vi "arrayToImage.vi"() -> ()   [LabVIEW 2011]
panel:
  in  "flip axis?":bool
  in  "fringe number":u32
  in  "Boolean":bool
  in  "yPixel":i32
  in  "xPixel":i32
  out "Image":T1(plugin-control)
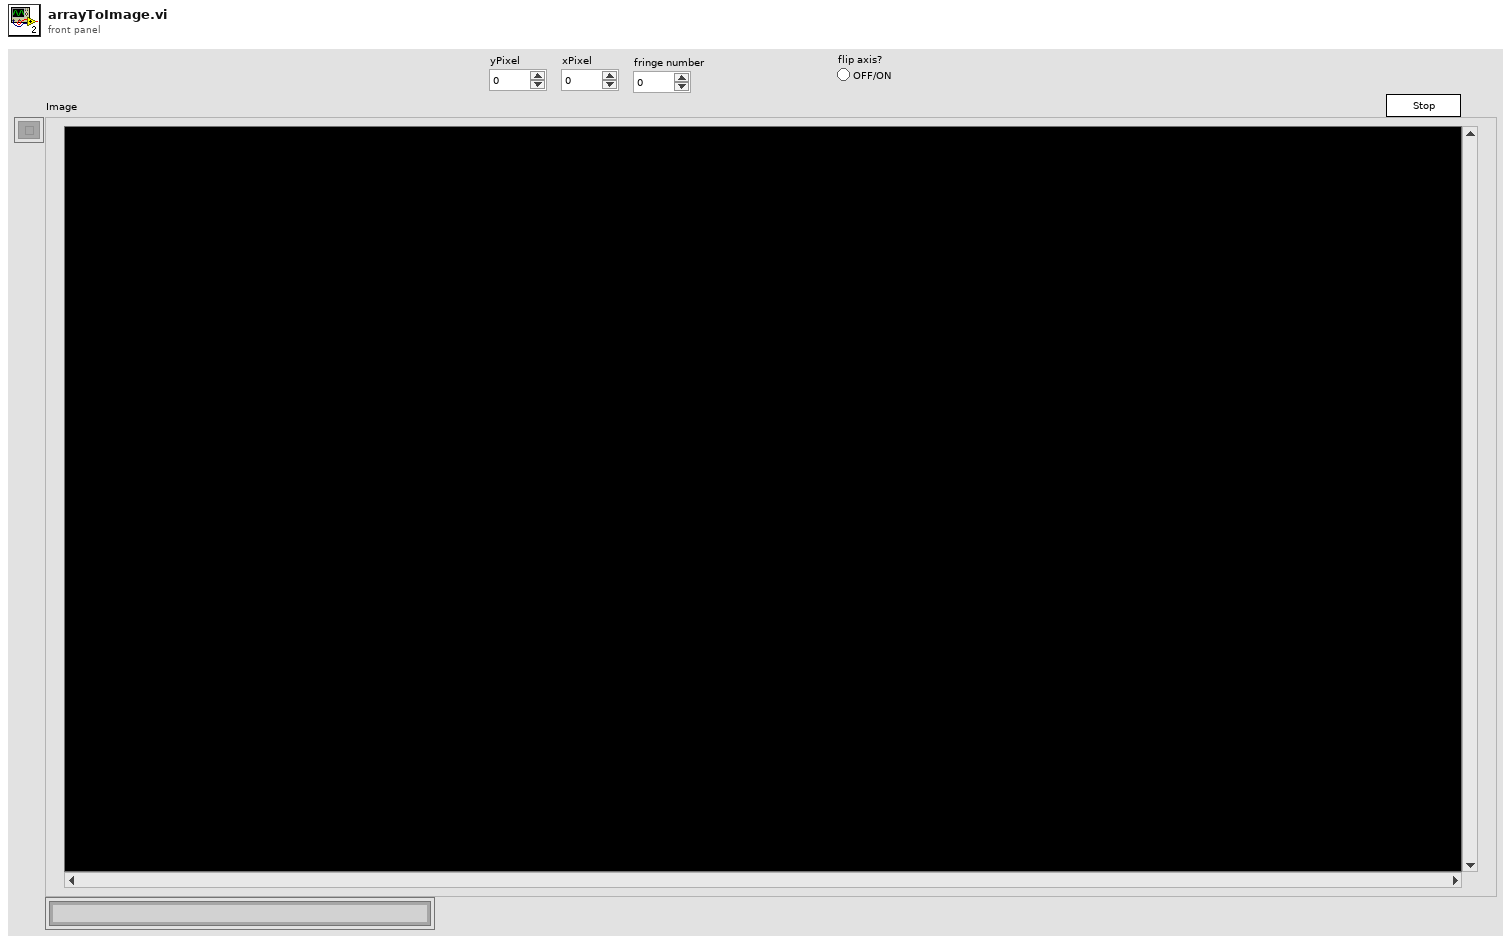
[diagram p1: front panel]
types:
  T1 = typedef "IMAQ Image.ctl" = refnum<image>
  T2 = typedef "Image Type" = u32
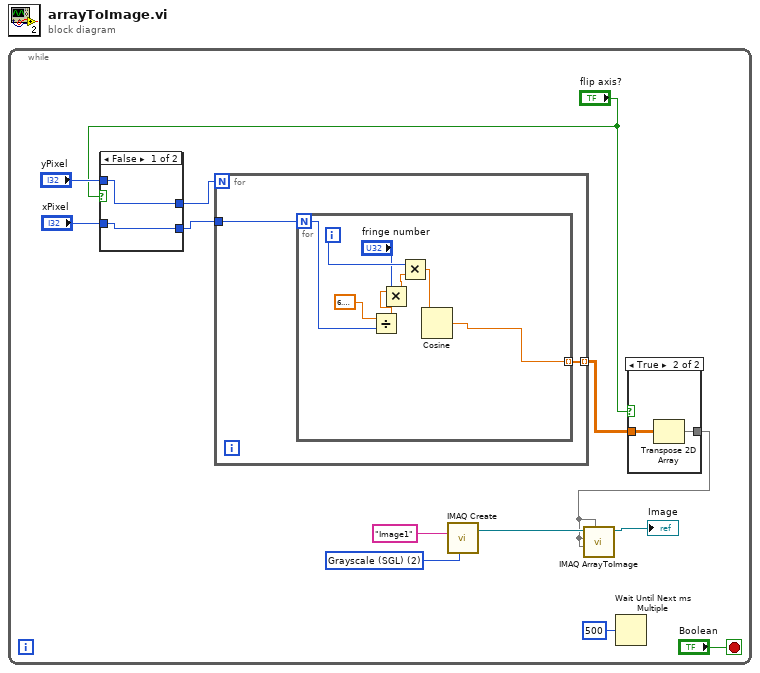
[diagram p0: block diagram]
diagram:
  n1 = while {
    stop <- "Boolean" stop-if-true
    w6 = T2 2 items=["Grayscale (U8)", "Grayscale (I16)", "Grayscale (SGL)", "Complex (CSG)", "RGB (U32)", "HSL (U32)", "RGB (U64)", "Grayscale (U16)"] ("Image Type")
    n2 = case shown="False" "flip axis?" {
      tunnel: "yPixel" -> [w15 w17]
      tunnel: "xPixel" -> [w14 w16]
      tunnel: [w14 w17] -> w3
      tunnel: [w15 w16] -> w2
      frame False {
      }
      frame True {
      }
    }
    n3 = for {
      N: w2 -> [_]
      tunnel: [w22] -> w8 mode=indexing
      tunnel: w3 -> [w21]
      n4 = for {
        N: w21 -> [w27]
        tunnel: [w23] -> w22 mode=indexing
        i -> [w29]
        n5 = Divide(x=6.283185307179586, y=w27) -> (x/y=w26:dbl)
        n6 = Multiply(x=w26, y="fringe number") -> (x*y=w25:dbl)
        n7 = Multiply(x=w29, y=w25) -> (x*y=w28:dbl)
        n8 = Cosine(x=w28) -> (cos(x)=w23:dbl)
      }
    }
    n9 = call "IMAQ Create"("Image Name"="Image1", "Image Type"=w6) -> ("New Image"=w12:T1)  [unwired: 2 in, 2 out]
    n10 = Wait Until Next ms Multiple(millisecond multiple=u32 500) -> ()  [unwired: 1 out]
    n11 = case shown="True" "flip axis?" {
      tunnel: w8 -> [w18 w20]
      tunnel: [w18 w19] -> w7
      frame False {
      }
      frame True {
        n12 = Transpose 2D Array(2D array=w20) -> (transposed array=w19:dbl[][])
      }
    }
    n13 = call "IMAQ ArrayToImage"("Image Pixels (Float)"=w7, "Image Pixels (U16)"=w7, "Image Pixels (I16)"=w7, "Image Pixels (U8)"=w7, "Image"=w12) -> ("Image Out"=→"Image":T1)  [unwired: 5 in, 1 out]
  }
